vi "Brute Force Measurment SubVI.vi"(0 "First Tube #":i32, 3 "Stop Program Brute Force":bool, 4 "Barcodes in":string[](array[string]), 5 "Channel # in":i32, 6 "Last Tube #":i32, 7 "error in (no error)":errorcluster, 9 "BoardHandle in":T1) -> (11 "Actual Voltage Level (V) 2":dbl format="%#_13g", 12 "Individual Tube Current (Nano Amps)":dbl[](array[numeric]), 13 "Failed Tubes":string[](array[string]), 18 "error out":errorcluster, 19 "BoardHandle out":T1)   [LabVIEW 2020]
panel:
  # "Pin in."
  # "Output pin positions"
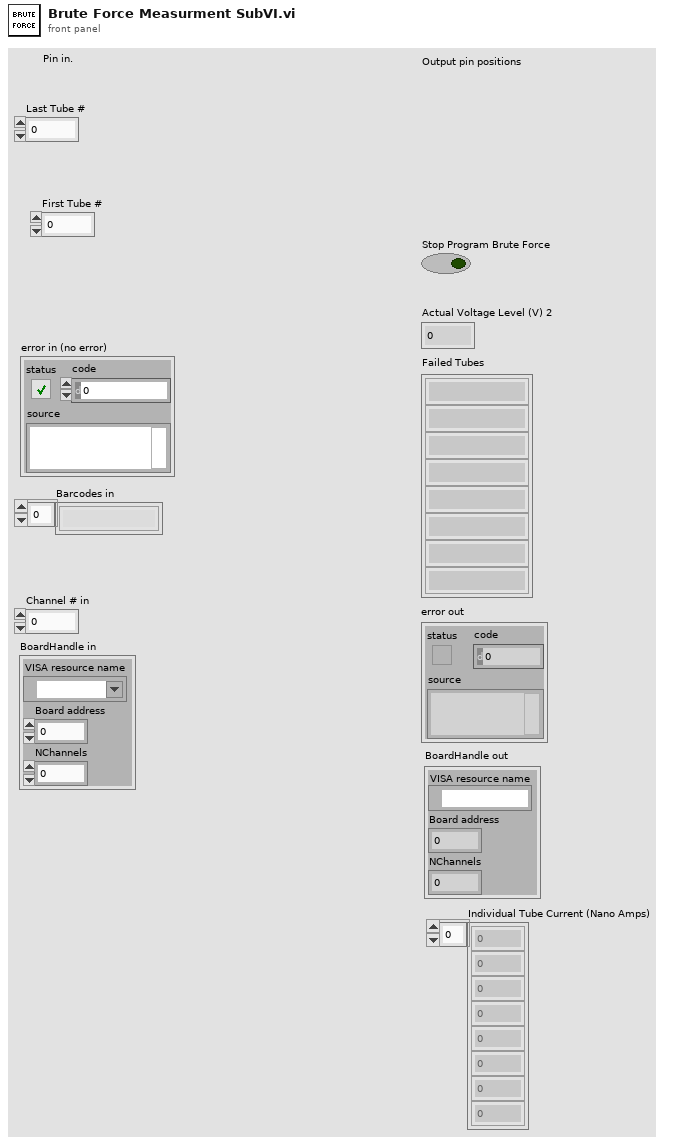
[diagram p1: front panel]
types:
  T1 = cluster{"VISA resource name":refnum<visa-resource-name>, "Board address":u8, "NChannels":u8}
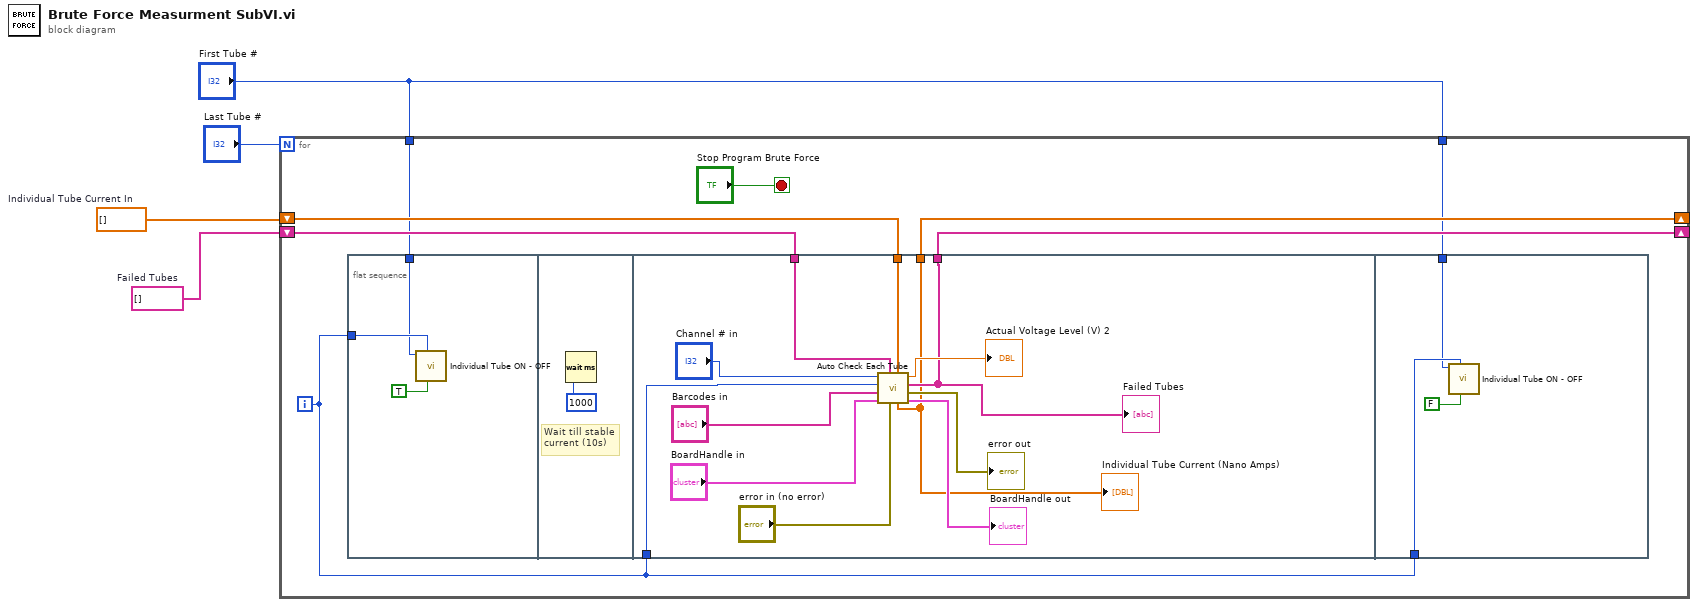
[diagram p0: block diagram]
diagram:
  w3 = dbl[] []  # Individual Tube Current In
  w4 = string[] []  # Failed Tubes
  n1 = for {
    N: "Last Tube #" -> [_]
    shift-right: [w10] -> _
    shift-left: w4 -> [w11]
    shift-right: [w8] -> _
    shift-left: w3 -> [w9]
    tunnel: "First Tube #" -> [w6]
    tunnel: "First Tube #" -> [w5]
    i -> [w12]
    stop <- "Stop Program Brute Force" stop-if-true
    n2 = flat-sequence {
      tunnel: w12 -> [w15]
      tunnel: w6 -> [w13]
      tunnel: w12 -> [w21]
      tunnel: w11 -> [w20]
      tunnel: [w19] -> w10
      tunnel: w9 -> [w18]
      tunnel: [w17] -> w8
      tunnel: w12 -> [w31]
      tunnel: w5 -> [w29]
      frame #0 {
        n3 = call "Individual Tube ON - OFF.vi"("Single Tube ON/OFF"=TRUE, "Tube #"=w15, "First Tube Number"=w13) -> ()  [unwired: 9 in]
      }
      frame #1 {
        # "Wait till stable\ncurrent (10s)"
        n4 = Wait (ms)(milliseconds to wait=u32 1000) -> ()  [unwired: 1 out]
      }
      frame #2 {
        n5 = call "Auto Check Each Tube.vi"("Individual Tube Current In"=w18, "error in (no error)"="error in (no error)", "Failed Tubes In"=w20, "BoardHandle in"="BoardHandle in", "Barcodes in"="Barcodes in", "Tube #"=w21, "Channel # in"="Channel # in") -> ("BoardHandle out"=→"BoardHandle out":T1, "error out"=→"error out":errorcluster, "Failed Tubes"=w19:string[], "Actual Voltage Level (V) 2"=→"Actual Voltage Level (V) 2":dbl, "Individual Tube Current (Nano Amps)"=w17:dbl[])
        "Failed Tubes" <- w19
        "Individual Tube Current (Nano Amps)" <- w17
      }
      frame #3 {
        n6 = call "Individual Tube ON - OFF.vi"("Single Tube ON/OFF"=FALSE, "Tube #"=w31, "First Tube Number"=w29) -> ()  [unwired: 9 in]
      }
    }
  }
